vi "Split Channel Data.vi"(0 "Input Array":u8[](array[numeric]), 11 "Error In":errorcluster) -> (4 "Channel 1 Data":u8[](array[numeric]), 6 "Channel 2 Data":u8[](array[numeric]), 8 "Channel 3 Data":u8[](array[numeric]), 10 "Channel 4 Data":u8[](array[numeric]), 15 "Error Out":errorcluster)   [LabVIEW 2021]
doc: "This VI splits the received 1D U8 array digital data of multiple channels based on the channel flags to respective channel U8 array."
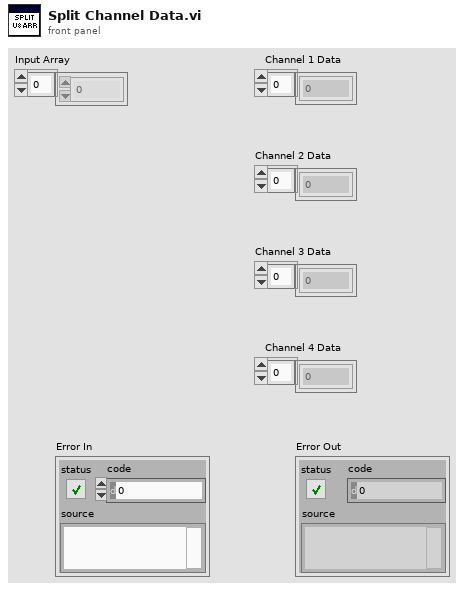
[diagram p1: front panel]
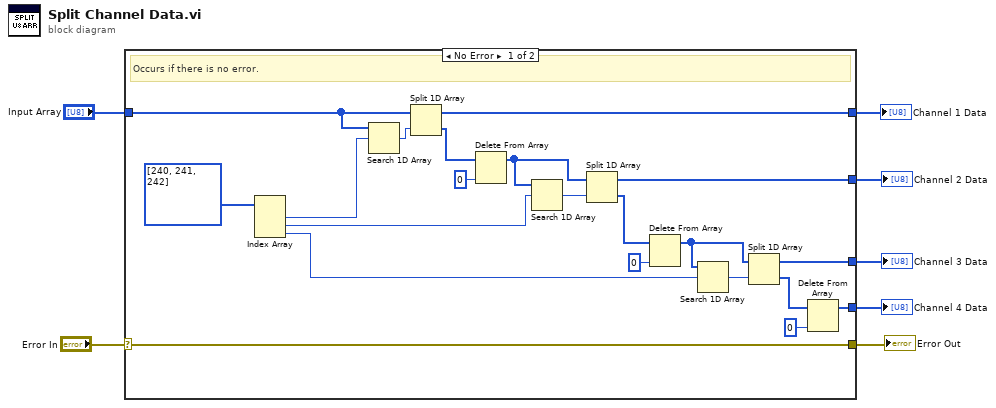
[diagram p0: block diagram]
diagram:
  n1 = case shown="No Error" "Error In" {
    selector: "Error In" -> [w8 w29]
    tunnel: "Input Array" -> [w26 _]
    tunnel: [w24 _] -> w6
    tunnel: [w18 _] -> w5
    tunnel: [w12 _] -> w4
    tunnel: [w9 _] -> w3
    tunnel: [w8 w29] -> w1
    frame No Error {
      # "Occurs if there is no error."
      n2 = Index Array(array=u8[] [240, 241, 242]) -> (element #1=w27:u8, element #2=w21:u8, element #3=w15:u8)  [unwired: 3 in]
      n3 = Search 1D Array(1D array=w26, element=w27) -> (index of element=w25:i32)  [unwired: 1 in]
      n4 = Split 1D Array(array=w26, index=w25) -> (first subarray=w24:u8[], second subarray=w23:u8[])
      n5 = Delete From Array(array=w23, index=0) -> (array with subset deleted=w19:u8[])  [unwired: 1 in, 1 out]
      n6 = Search 1D Array(1D array=w19, element=w21) -> (index of element=w20:i32)  [unwired: 1 in]
      n7 = Split 1D Array(array=w19, index=w20) -> (first subarray=w18:u8[], second subarray=w17:u8[])
      n8 = Delete From Array(array=w17, index=0) -> (array with subset deleted=w13:u8[])  [unwired: 1 in, 1 out]
      n9 = Search 1D Array(1D array=w13, element=w15) -> (index of element=w14:i32)  [unwired: 1 in]
      n10 = Split 1D Array(array=w13, index=w14) -> (first subarray=w12:u8[], second subarray=w11:u8[])
      n11 = Delete From Array(array=w11, index=0) -> (array with subset deleted=w9:u8[])  [unwired: 1 in, 1 out]
    }
    frame Error {
      # "Occurs if there is any error."
    }
  }
  "Channel 1 Data" <- w6
  "Channel 2 Data" <- w5
  "Channel 3 Data" <- w4
  "Channel 4 Data" <- w3
  "Error Out" <- w1
